vi "slopes2zern2diff_test_old.vi"() -> ()   [LabVIEW 2018]
uses:
  <userlib>/WaveKit.lib/Controls/HasoSlopes.lvclass
panel:
  in  "Hasao slopes file 2":path=path "D:/Data/20200627_AbeComponentCheck/ZernIdx_1_0.has"
  in  "Output folder":path=path "D:/Data/20200627_AbeComponentCheck"
  in  "Output file base name":string="ZernIdx_1_diff.txt"
  in  "Hasao slopes file 1":path=path "D:/Data/20200627_AbeComponentCheck/ZernIdx_1.has"
  out "Zernike pupil":i32[][](graph)
  out "Measured pupil":i32[][](graph)
  out "Diff of Zernike Coefficients":sgl[](graph)
  out "error out":errorcluster
  # "Convert two slopes to Zernike coeffs and calculate the difference: slopes1 - slopes2"
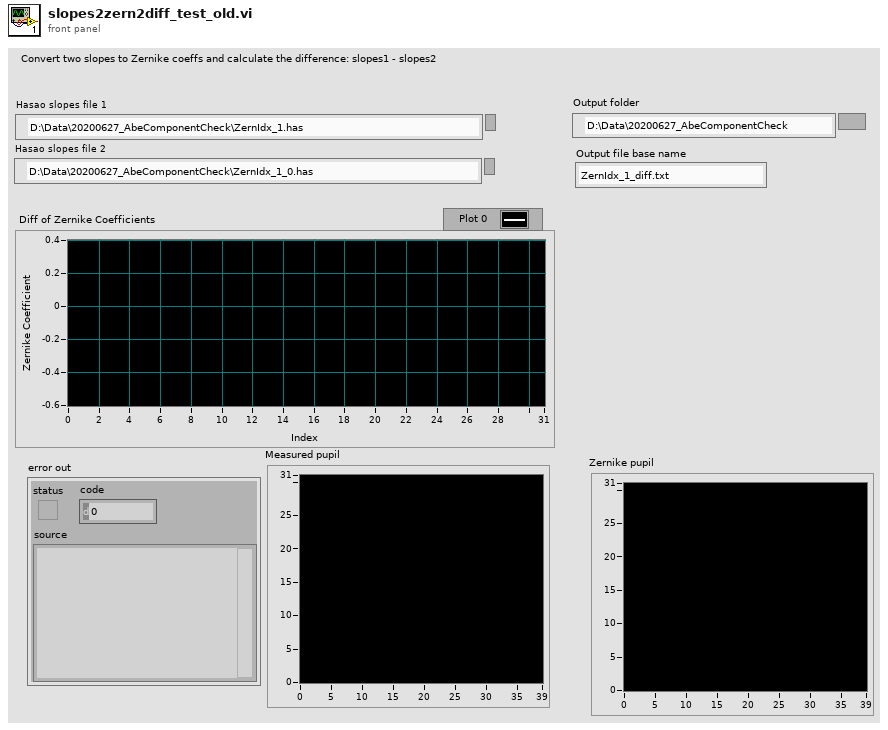
[diagram p1: front panel]
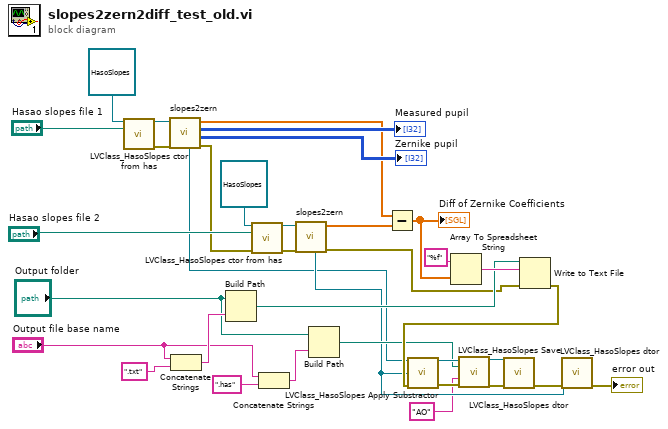
[diagram p0: block diagram]
diagram:
  n1 = call <userlib>:"LVClass_HasoSlopes ctor from has.vi"("HasoSlopes in"=refnum<class "HasoSlopes.lvclass"> refnum, ".has path"="Hasao slopes file 1") -> ("HasoSlopes out"=w27:refnum<class "HasoSlopes.lvclass">, "error out"=w28:errorcluster)  [unwired: 12 in]
  n2 = call "slopes2zern.vi"("HasoSlopes in"=w27, "error in (no error)"=w28) -> ("HasoSlopes out"=w2:refnum<class "HasoSlopes.lvclass">, "Zernike Coefficients"=w21:sgl[], "Measured pupil"=→"Measured pupil":i32[][], "Zernike pupil"=→"Zernike pupil":i32[][], "error out"=w24:errorcluster)  [unwired: 4 in]
  n3 = Concatenate Strings("Output file base name", ".txt") -> (w17:string)
  n4 = Build Path(base path="Output folder", name or relative path=w17) -> (appended path=w31:path)
  n5 = call <userlib>:"LVClass_HasoSlopes ctor from has.vi"("HasoSlopes in"=refnum<class "HasoSlopes.lvclass"> refnum, ".has path"="Hasao slopes file 2", "error in (no error)"=w24) -> ("HasoSlopes out"=w23:refnum<class "HasoSlopes.lvclass">, "error out"=w22:errorcluster)  [unwired: 11 in]
  n6 = Concatenate Strings("Output file base name", ".has") -> (w15:string)
  n7 = call "slopes2zern.vi"("HasoSlopes in"=w23, "error in (no error)"=w22) -> ("HasoSlopes out"=w3:refnum<class "HasoSlopes.lvclass">, "Zernike Coefficients"=w20:sgl[], "error out"=w7:errorcluster)  [unwired: 4 in, 2 out]
  n8 = Build Path(base path="Output folder", name or relative path=w15) -> (appended path=w4:path)
  n9 = Subtract(x=w21, y=w20) -> (x-y=w19:sgl[])
  "Diff of Zernike Coefficients" <- w19
  n10 = Array To Spreadsheet String(array=w19, 3:"%f") -> (spreadsheet string=w32:string)  [unwired: 1 in]
  n11 = Write to Text File(file (use dialog)=w31, text=w32, error in=w7) -> (error out=w6:errorcluster)  [unwired: 1 in, 2 out]
  n12 = call <userlib>:"LVClass_HasoSlopes Apply Substractor.vi"("HasoSlopes in"=w2, "HasoSlopes to substract"=w3, "error in (no error)"=w6) -> ("HasoSlopes out"=w12:refnum<class "HasoSlopes.lvclass">, "error out"=w8:errorcluster)  [unwired: 11 in]
  n13 = call <userlib>:"LVClass_HasoSlopes Save.vi"("HasoSlopes in"=w12, "path"=w4, "session"="AO", "error in (no error)"=w8) -> ("HasoSlopes out"=w11:refnum<class "HasoSlopes.lvclass">, "error out"=w9:errorcluster)  [unwired: 10 in]
  n14 = call <userlib>:"LVClass_HasoSlopes dtor.vi"("HasoSlopes in"=w11, "error in (no error)"=w9) -> ("error out"=w10:errorcluster)  [unwired: 12 in, 1 out]
  n15 = call <userlib>:"LVClass_HasoSlopes dtor.vi"("HasoSlopes in"=w3, "error in (no error)"=w10) -> ("error out"=→"error out":errorcluster)  [unwired: 12 in, 1 out]
